vi "Run Tests Programmatically.vi"(4 "Verbose":bool=TRUE, 5 "Silent":bool, 6 "Interactive":bool=TRUE, 7 "Inspect Recursively":bool=TRUE, 9 "Report name":string, 10 "Output Folder":path, 11 "Source Folder":path) -> ()   [LabVIEW 2013]
uses:
  classes/Test Runner/Test Runner.lvclass
  classes/Test Runner/Test Runner.lvclass/Test Runner.ctl
  <userlib>/_OpenG.lib/file/file.llb/Valid Path - Traditional__ogtk.vi
  <userlib>/_OpenG.lib/file/file.llb/File Exists - Scalar__ogtk.vi
  <userlib>/_OpenG.lib/array/array.llb/Delete Elements from 1D Array (Path)__ogtk.vi
  <userlib>/_OpenG.lib/file/file.llb/Strip Path - Arrays__ogtk.vi
  <userlib>/_OpenG.lib/file/file.llb/Strip Path Extension - 1D Array of Strings__ogtk.vi
  <userlib>/_OpenG.lib/file/file.llb/Strip Path Extension - String__ogtk.vi
  <userlib>/_OpenG.lib/file/file.llb/Convert File Extension (String)__ogtk.vi
  classes/Test Report.JUnit/Test Report.JUnit.lvclass
  classes/Test Report.Default/Test Report.Default.lvclass
panel:
  in  "report format":enum16{"Plain text", "XML"}(ring)=enum."XML"
  in  "Defined Tests":i32[](listbox)
  in  "Run Batch Test":bool
  # "CARAYA Batch Testing\n\nFill in the source folder where your tests are and choose the output result options."
  # "Output Configuration"
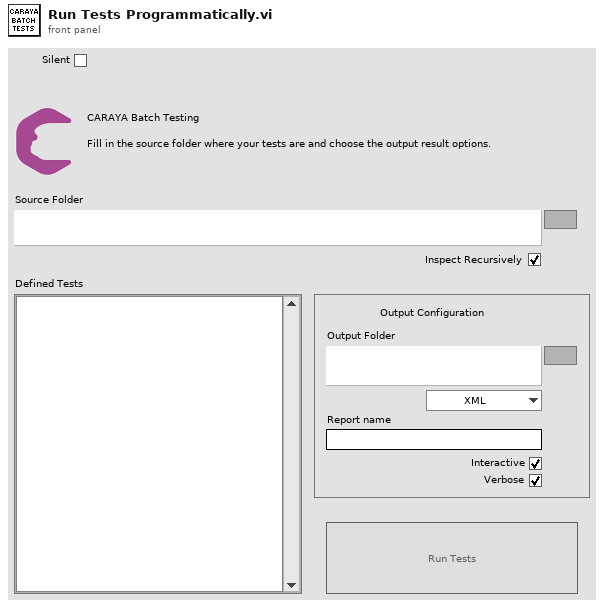
[diagram p1: front panel]
types:
  T1 = enum32{"invalid app kind", "Development System", "Run Time System", "Student Edition", "Embedded LabVIEW", "Evaluation", "Custom"}
  T2 = enum8{"Enabled", "Disabled", "Disabled and Grayed Out"}
  T3 = enum32{"Invalid", "Standard", "Closed", "Hidden", "Minimized", "Maximized"}
  T4 = cluster{"Core":cluster{"Current VI Reference":refnum<vi>, "Close Panel on Exit?":bool}, "Output Folder":path, "Report name":string, "Source Folder":path, "Interactive":bool, "Verbose":bool, "Menu Launch AppRef":refnum<vi>, "Silent":bool, "report format":enum16{"Plain text", "XML"}, "Test Runner":refnum<class "Test Runner.lvclass">}
  T5 = cluster{"Current VI Reference":refnum<vi>, "Close Panel on Exit?":bool}
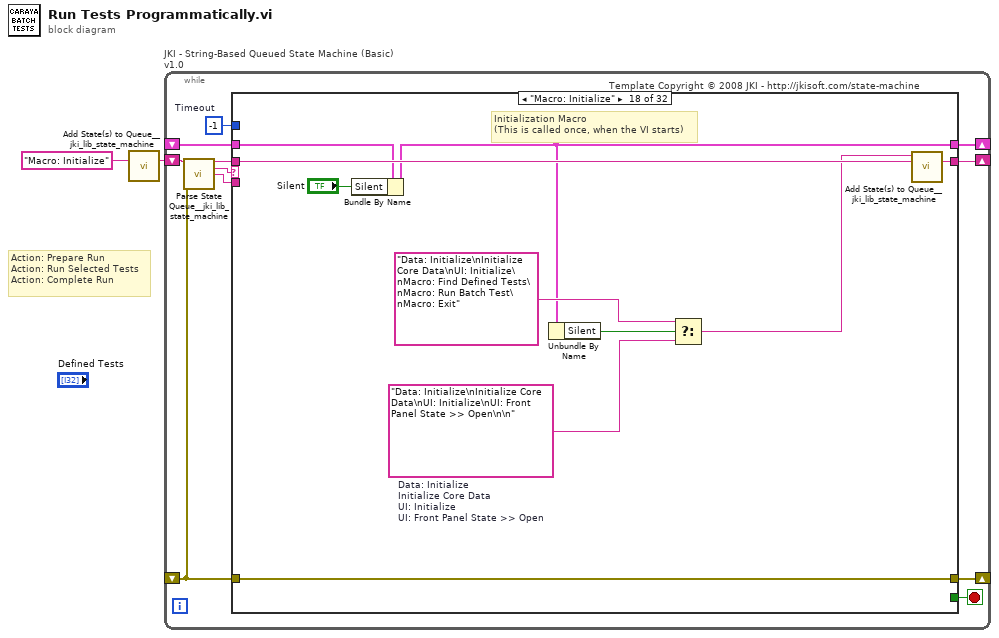
[diagram p0: block diagram]
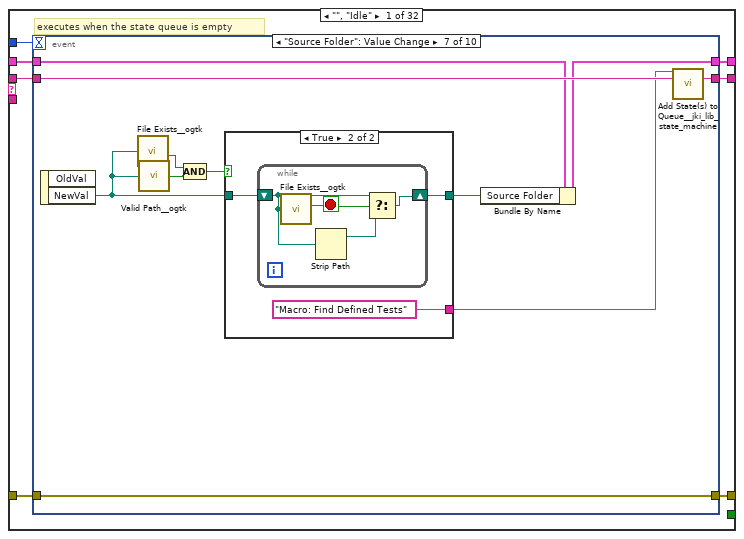
[diagram p2: hidden frame]
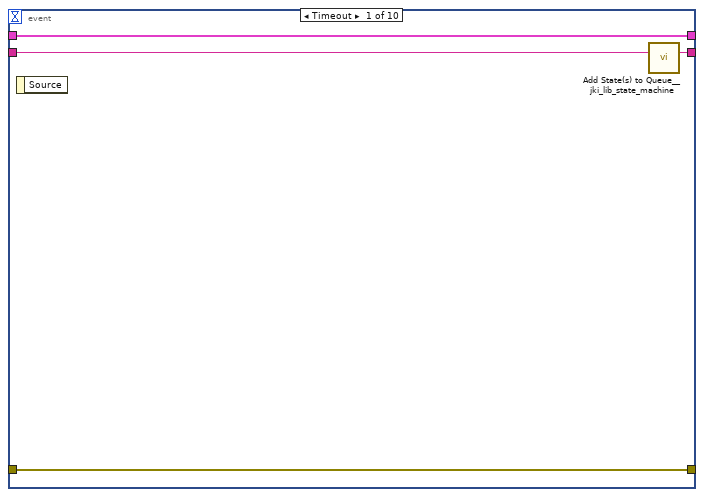
[diagram p3: hidden frame]
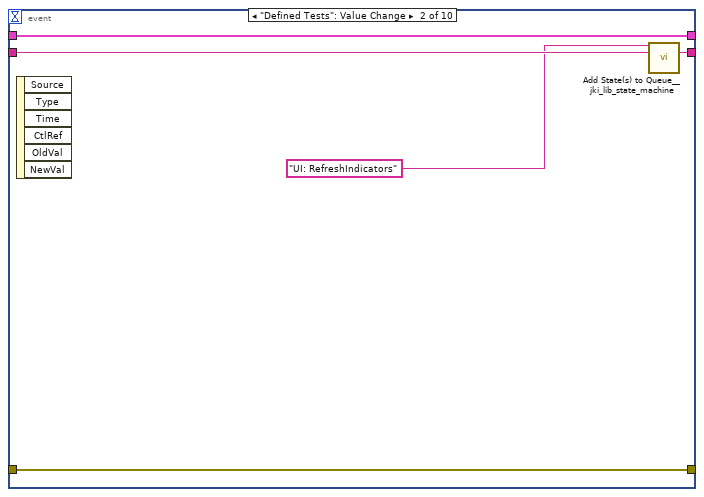
[diagram p4: hidden frame]
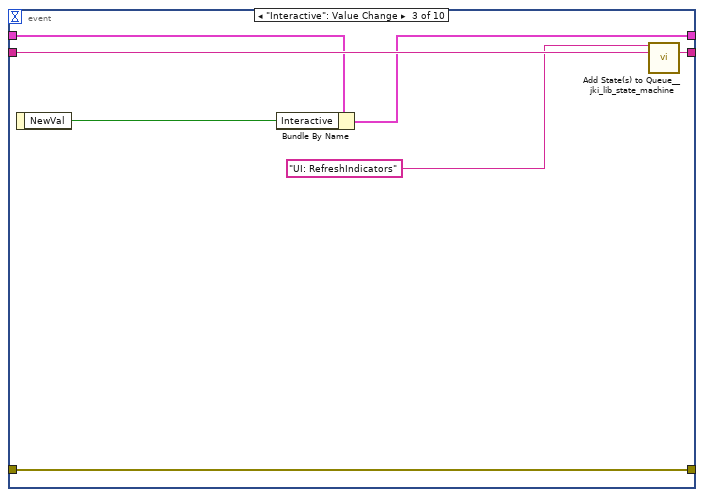
[diagram p5: hidden frame]
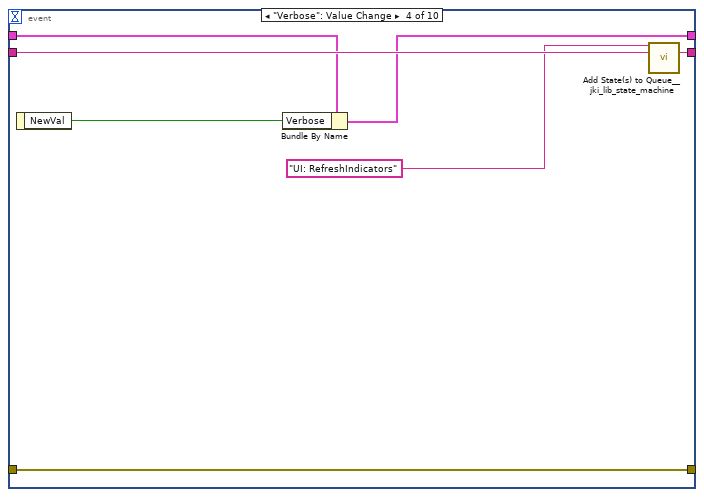
[diagram p6: hidden frame]
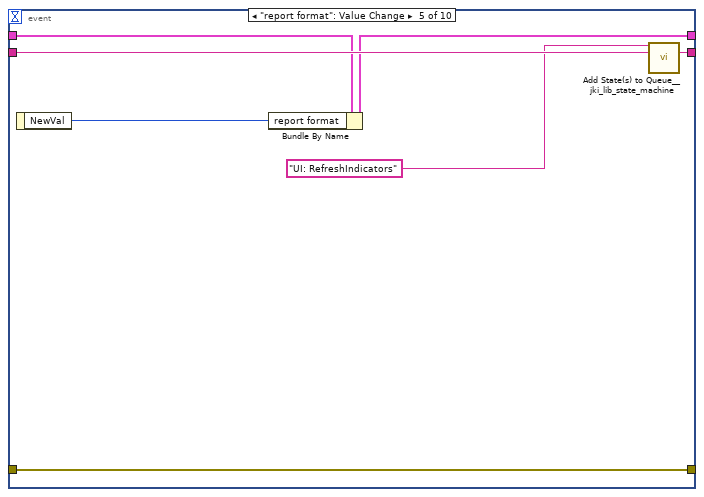
[diagram p7: hidden frame]
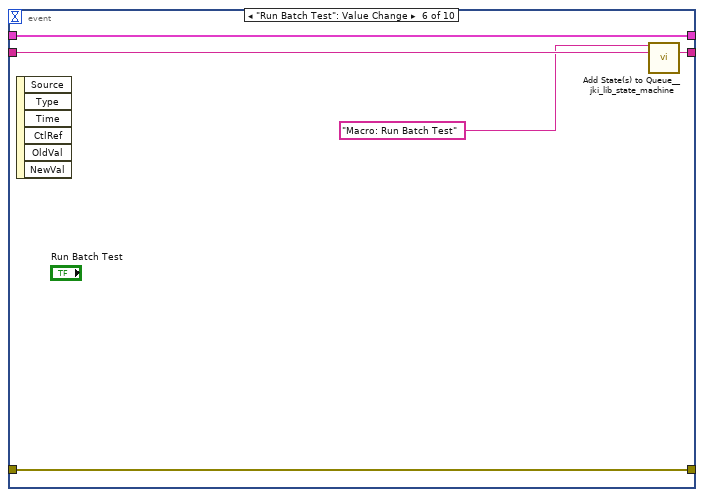
[diagram p8: hidden frame]
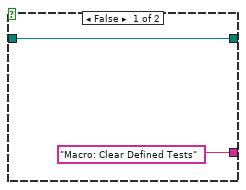
[diagram p9: hidden frame]
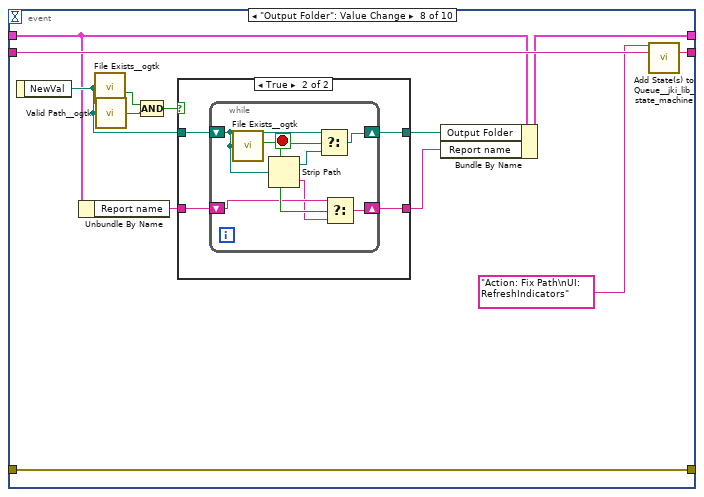
[diagram p10: hidden frame]
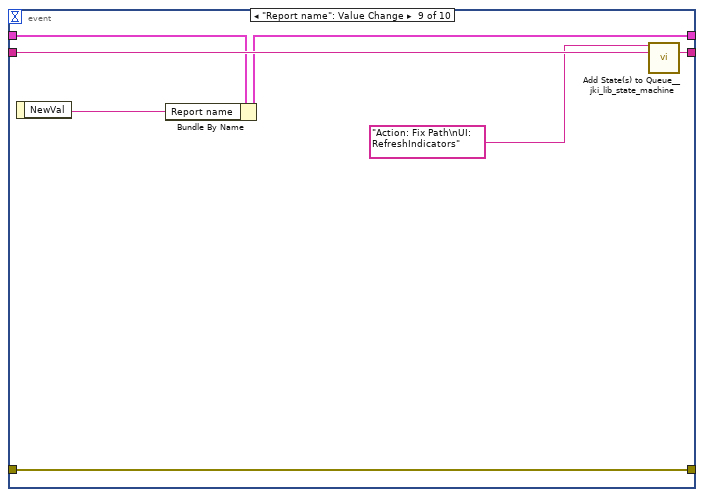
[diagram p12: hidden frame]
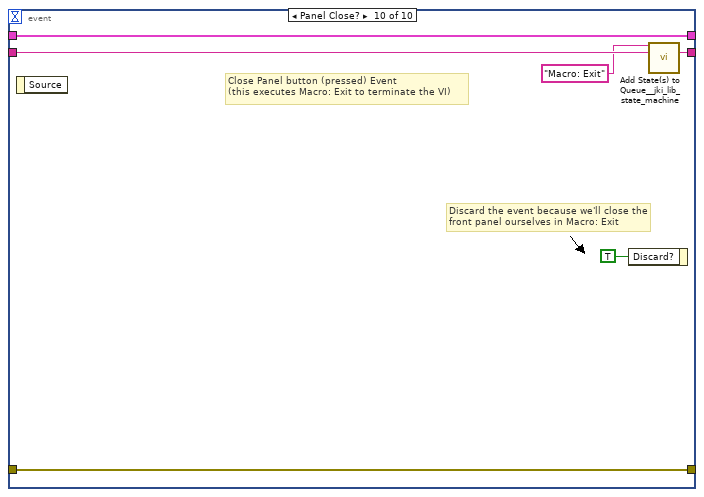
[diagram p13: hidden frame]
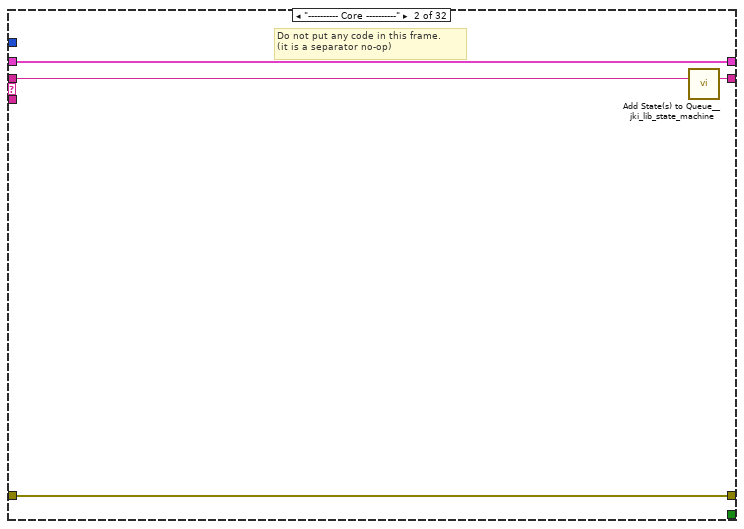
[diagram p14: hidden frame]
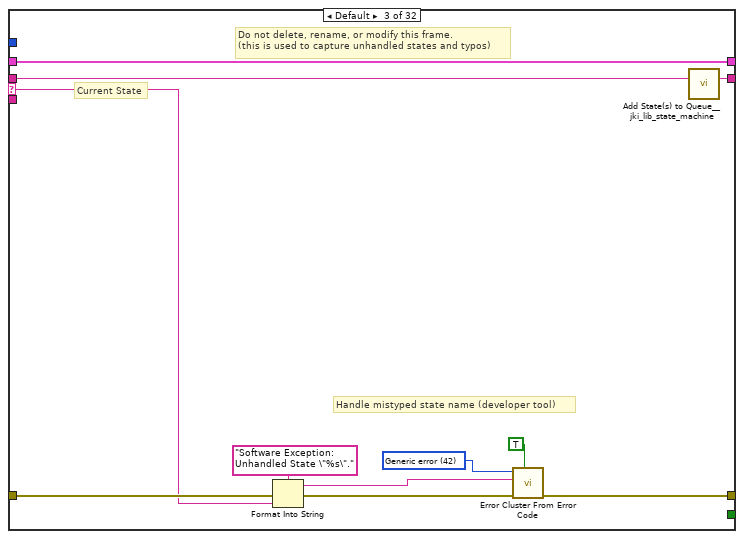
[diagram p15: hidden frame]
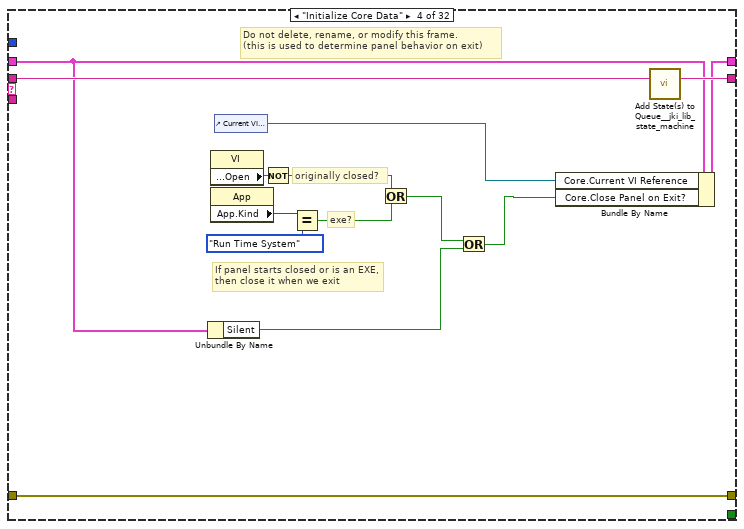
[diagram p16: hidden frame]
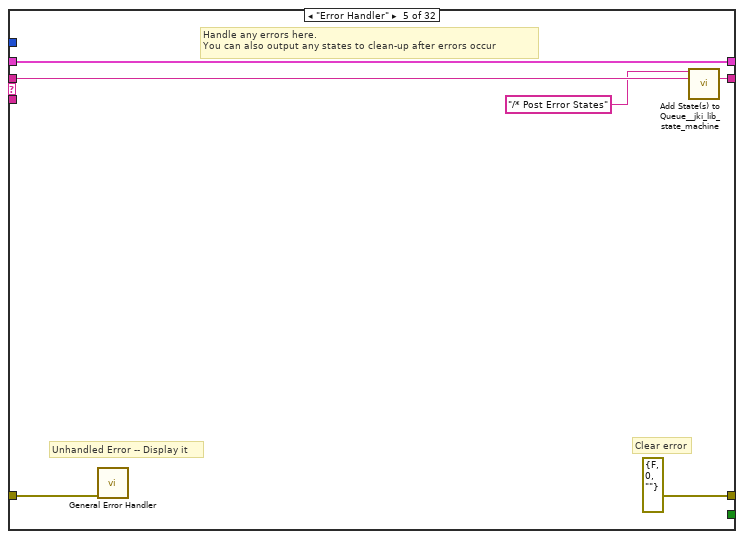
[diagram p17: hidden frame]
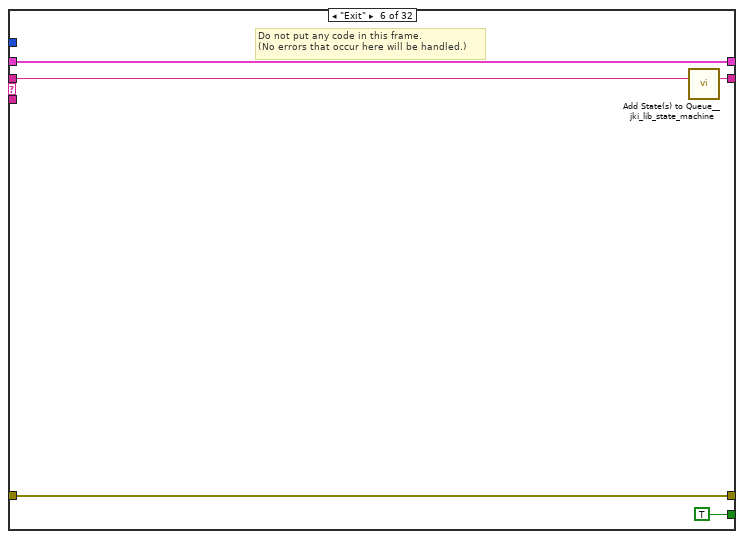
[diagram p18: hidden frame]
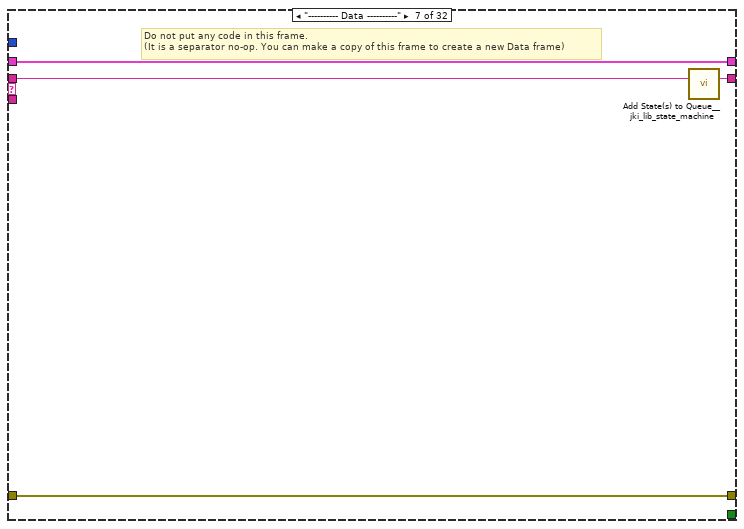
[diagram p19: hidden frame]
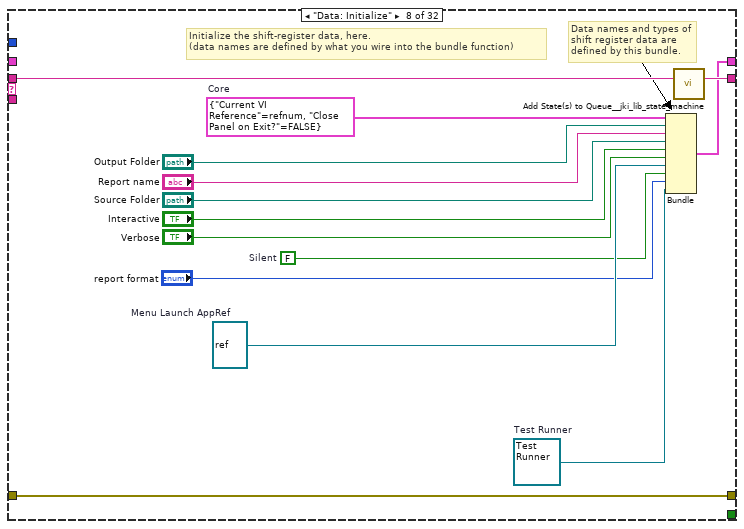
[diagram p20: hidden frame]
diagram:
  # "Action: Prepare Run\nAction: Run Selected Tests\nAction: Complete Run"
  n1 = call <vilib>:"Add State(s) to Queue__jki_lib_state_machine.vi"("State(s) in (\"\")"="Macro: Initialize") -> ("States Out"=w2:string)  [unwired: 14 in]
  n2 = while "JKI - String-Based Queued State Machine (Basic) v1.0" {
    shift-right: [w6] -> _
    shift-left: _ -> [w5]
    shift-right: [w9] -> _
    shift-left: _ -> [w3]
    shift-right: [w8] -> _
    shift-left: w2 -> [w10]
    stop <- w7 stop-if-true
    w4 = -1  # Timeout
    # "Template Copyright © 2008 JKI - http://jkisoft.com/state-machine"
    n3 = call <vilib>:"Parse State Queue__jki_lib_state_machine.vi"("State Queue"=w10, "Error In (no error)"=w3) -> ("Remaining States"=w12:string, "Current State"=w13:string, "Arguments"=w11:string)  [unwired: 11 in]
    n4 = case shown="\"Macro: Initialize\"" w13 {
      selector: w13 -> [_ _ w119 _ _ _ _ _ _ _ _ _ _ _ _ _ _ _ _ _ _ _ _ _ _ _ _ _ _ _ _ _]
      tunnel: w12 -> [w20 w118 w123 w143 w149 w154 w158 w172 w178 w182 w191 w221 w240 w251 w260 w271 w297 w307 w312 w317 w322 w327 w332 w339 w343 w361 w396 w407 w421 w428 w447 w467]
      tunnel: w11 -> [_ _ _ _ _ _ _ _ _ _ _ _ _ _ w255 w265 _ _ _ _ _ _ _ _ _ _ _ _ _ _ _ _]
      tunnel: w5 -> [w18 w115 w121 w133 w146 w152 w155 _ w173 w179 w187 w215 w238 w249 w258 w267 w294 w301 w309 w314 w319 w324 w329 w336 w340 w358 w394 w405 w415 w425 w435 w464]
      tunnel: [w17 w116 w125 w140 errorcluster {"status"=FALSE, "code"=0, "source"=""} ("error out") w151 w156 w169 w174 w180 w189 w219 w224 w244 w256 w268 w295 w305 w310 w315 w320 w325 w330 w337 w341 w359 w386 w397 w418 w426 w439 w465] -> w9
      tunnel: w3 -> [w16 w116 w124 w140 w145 w151 w156 w169 w175 w180 w189 w219 w224 w245 w257 w269 w295 w305 w310 w315 w320 w325 w330 w337 w341 w359 w387 w398 w419 w426 w440 w465]
      tunnel: [w19 w117 w122 w142 w148 w153 w157 w171 w177 w181 w190 w220 w239 w250 w259 w270 w296 w306 w311 w316 w321 w326 w331 w338 w342 w360 w395 w406 w420 w427 w446 w466] -> w8
      tunnel: [_ _ _ _ _ TRUE _ _ _ _ _ _ _ _ _ _ _ _ _ _ _ _ _ _ _ _ _ _ _ _ _ _] -> w7
      tunnel: [w15 w115 w121 w141 w146 w152 w155 w170 w173 w179 w186 w214 w237 w249 w258 w267 w294 w300 w309 w314 w319 w324 w329 w336 w340 w352 w393 w404 w414 w425 w441 w464] -> w6
      tunnel: w4 -> [w14 _ _ _ _ _ _ _ _ _ _ _ _ _ _ _ _ _ _ _ _ _ _ _ _ _ _ _ _ _ _ _]
      frame "", "Idle" {
        # "executes when the state queue is empty"
        n5 = event shown="[6] \"Source Folder\": Value Change" {
          selector: _ -> [_ _ _ _ _ _ _ _ _ _]
          dyn-events: _ -> [_ _ _ _ _ _ _ _ _ _]
          timeout: w14 -> [_ _ _ _ _ _ _ _ _ _]
          tunnel: w20 -> [w24 w29 w36 w43 w50 w55 w66 w88 w108 w114]
          tunnel: [w23 w28 w35 w42 w49 w54 w65 w87 w107 w113] -> w19
          tunnel: w18 -> [w21 w26 w31 w38 w45 w52 w63 w78 w105 w111]
          tunnel: [w22 w27 w34 w41 w48 w53 w64 w86 w106 w112] -> w17
          tunnel: w16 -> [w22 w27 w34 w41 w48 w53 w64 w86 w106 w112]
          tunnel: [w21 w26 w30 w37 w44 w52 w62 w85 w104 w111] -> w15
          event Timeout {
            n6 = event-data() -> ()  [unwired: 1 in, 1 out]
            n7 = call <vilib>:"Add State(s) to Queue__jki_lib_state_machine.vi"("State(s) in (\"\")"=w24) -> ("States Out"=w23:string)  [unwired: 14 in]
          }
          event "Defined Tests": Value Change {
            n8 = event-data() -> ()  [unwired: 1 in, 6 out]
            n9 = call <vilib>:"Add State(s) to Queue__jki_lib_state_machine.vi"("State(s) in Front (\"\")"="UI: RefreshIndicators", "State(s) in (\"\")"=w29) -> ("States Out"=w28:string)  [unwired: 13 in]
          }
          event "Interactive": Value Change {
            n10 = event-data() -> ("NewVal"=w32:bool)  [unwired: 1 in]
            n11 = Bundle By Name(cluster=w31, "Interactive"=w32) -> (w30:T4)
            n12 = call <vilib>:"Add State(s) to Queue__jki_lib_state_machine.vi"("State(s) in Front (\"\")"="UI: RefreshIndicators", "State(s) in (\"\")"=w36) -> ("States Out"=w35:string)  [unwired: 13 in]
          }
          event "Verbose": Value Change {
            n13 = event-data() -> ("NewVal"=w39:bool)  [unwired: 1 in]
            n14 = Bundle By Name(cluster=w38, "Verbose"=w39) -> (w37:T4)
            n15 = call <vilib>:"Add State(s) to Queue__jki_lib_state_machine.vi"("State(s) in Front (\"\")"="UI: RefreshIndicators", "State(s) in (\"\")"=w43) -> ("States Out"=w42:string)  [unwired: 13 in]
          }
          event "report format": Value Change {
            n16 = event-data() -> ("NewVal"=w46:enum16{"Plain text", "XML"})  [unwired: 1 in]
            n17 = Bundle By Name(cluster=w45, "report format"=w46) -> (w44:T4)
            n18 = call <vilib>:"Add State(s) to Queue__jki_lib_state_machine.vi"("State(s) in Front (\"\")"="UI: RefreshIndicators", "State(s) in (\"\")"=w50) -> ("States Out"=w49:string)  [unwired: 13 in]
          }
          event "Run Batch Test": Value Change {
            n19 = event-data() -> ()  [unwired: 1 in, 6 out]
            n20 = call <vilib>:"Add State(s) to Queue__jki_lib_state_machine.vi"("State(s) in Front (\"\")"="Macro: Run Batch Test", "State(s) in (\"\")"=w55) -> ("States Out"=w54:string)  [unwired: 13 in]
          }
          event "Source Folder": Value Change {
            n21 = event-data() -> ("NewVal"=w58:path)  [unwired: 1 in, 1 out]
            n22 = call-poly <userlib>:"File Exists__ogtk.vi"("file path"=w58) -> ("exists"=w60:bool)  [unwired: 6 in, 1 out]
            n23 = call-poly <userlib>:"Valid Path__ogtk.vi"("path"=w58) -> ("valid"=w61:bool)
            n24 = Compound Arithmetic op=AND(w60, w61) -> (w59:bool)
            n25 = case shown="True" w59 {
              tunnel: w58 -> [w68 w71]
              tunnel: [w68 w70] -> w57
              tunnel: ["Macro: Clear Defined Tests" "Macro: Find Defined Tests"] -> w56
              frame False {
              }
              frame True {
                n26 = while {
                  shift-right: [w74] -> w70
                  shift-left: w71 -> [w73]
                  stop <- w75 stop-if-true
                  n27 = call-poly <userlib>:"File Exists__ogtk.vi"("file path"=w73) -> ("is directory"=w75:bool)  [unwired: 6 in, 1 out]
                  n28 = Strip Path(path=w73) -> (stripped path=w72:path)  [unwired: 1 out]
                  n29 = Select(t=w73, s=w75, f=w72) -> (s? t:f=w74:path)
                }
              }
            }
            n30 = Bundle By Name(cluster=w63, "Source Folder"=w57) -> (w62:T4)
            n31 = call <vilib>:"Add State(s) to Queue__jki_lib_state_machine.vi"("State(s) in Front (\"\")"=w56, "State(s) in (\"\")"=w66) -> ("States Out"=w65:string)  [unwired: 13 in]
          }
          event "Output Folder": Value Change {
            n32 = event-data() -> ("NewVal"=w81:path)  [unwired: 1 in]
            n33 = Unbundle By Name(w78) -> ("Report name"=w77:string)
            n34 = call-poly <userlib>:"File Exists__ogtk.vi"("file path"=w81) -> ("exists"=w83:bool)  [unwired: 6 in, 1 out]
            n35 = call-poly <userlib>:"Valid Path__ogtk.vi"("path"=w81) -> ("valid"=w84:bool)
            n36 = Compound Arithmetic op=AND(w83, w84) -> (w82:bool)
            n37 = case shown="True" w82 {
              tunnel: w81 -> [w90 w94]
              tunnel: [w90 w93] -> w80
              tunnel: w77 -> [w89 w92]
              tunnel: [w89 w91] -> w76
              frame False {
              }
              frame True {
                n38 = while {
                  shift-right: [w101] -> w93
                  shift-left: w94 -> [w100]
                  shift-right: [w95] -> w91
                  shift-left: w92 -> [w97]
                  stop <- w98 stop-if-true
                  n39 = call-poly <userlib>:"File Exists__ogtk.vi"("file path"=w100) -> ("is directory"=w98:bool)  [unwired: 6 in, 1 out]
                  n40 = Strip Path(path=w100) -> (stripped path=w99:path, name=w96:string)
                  n41 = Select(t=w100, s=w98, f=w99) -> (s? t:f=w101:path)
                  n42 = Select(t=w97, s=w98, f=w96) -> (s? t:f=w95:string)
                }
              }
            }
            n43 = Bundle By Name(cluster=w78, "Output Folder"=w80, "Report name"=w76) -> (w85:T4)
            n44 = call <vilib>:"Add State(s) to Queue__jki_lib_state_machine.vi"("State(s) in Front (\"\")"="Action: Fix Path\nUI: RefreshIndicators", "State(s) in (\"\")"=w88) -> ("States Out"=w87:string)  [unwired: 13 in]
          }
          event "Report name": Value Change {
            n45 = event-data() -> ("NewVal"=w103:string)  [unwired: 1 in]
            n46 = Bundle By Name(cluster=w105, "Report name"=w103) -> (w104:T4)
            n47 = call <vilib>:"Add State(s) to Queue__jki_lib_state_machine.vi"("State(s) in Front (\"\")"="Action: Fix Path\nUI: RefreshIndicators", "State(s) in (\"\")"=w108) -> ("States Out"=w107:string)  [unwired: 13 in]
          }
          event Panel Close? {
            # "Discard the event because we'll close the front panel ourselves in Macro: Exit"
            # "Close Panel button (pressed) Event\n(this executes Macro: Exit to terminate the VI)"
            n48 = event-data() -> ()  [unwired: 1 in, 1 out]
            n49 = event-data("Discard?"=TRUE) -> ()  [unwired: 1 in, 1 out]
            n50 = call <vilib>:"Add State(s) to Queue__jki_lib_state_machine.vi"("State(s) in Front (\"\")"="Macro: Exit", "State(s) in (\"\")"=w114) -> ("States Out"=w113:string)  [unwired: 13 in]
          }
        }
      }
      frame "---------- Core ----------" {
        # "Do not put any code in this frame.\n(it is a separator no-op)"
        n51 = call <vilib>:"Add State(s) to Queue__jki_lib_state_machine.vi"("State(s) in (\"\")"=w118) -> ("States Out"=w117:string)  [unwired: 14 in]
      }
      frame Default {
        w128 = 42 items=["No error", "Argument error", "Memory is full", "Out of zone", "End of file", "File already open", "Generic file I/O error", "File not found", "File permission error", "Disk is full", "Duplicate path", "Too many files open", "System feature not enabled", "Resource file not found", "Cannot add resource", "Resource not found", "Image not found", "Image memory error", "Pen does not exist", "Config type invalid", "Config token not found", "Config parse error", "Config memory error", "Bad external code format", "Bad external code offset", "External code not present", "Null window", "Destroy window error", "Null menu", "Print aborted", "Bad print record", "Print driver error", "Windows error during printing", "Memory error during printing", "Print dialog error", "Generic print error", "Invalid device refnum", "Device not found", "Device parameter error", "Device unit error", "Cannot open device", "Device call aborted", "Generic error", "Cancelled by user", "Object ID too low", "Object ID too high", "Object not in heap", "Unknown heap", "Unknown object (invalid DefProc)", "Unknown object (DefProc not in table)", "Message out of range", "Invalid (null) method", "Unknown message", "Manager call not supported", "Bad address", "Network operation in progress", "Network operation timed out", "Connection is busy", "Network attribute not supported", "Network error", "Address in use", "System out of memory", "Connection aborted", "Connection refused", "Not connected", "Already connected", "Connection closed", "Initialization error (interapplication manager)", "Bad occurrence", "Wait on unbound occurrence handler", "Occurrence queue overflow", "Datalog type conflict", "Unused", "Unrecognized type (interapplication manager)", "Memory corrupt", "Failed to make temporary DLL", "Old CIN version", "Drag socket not found", "Failed to load drop-object", "Failed to register OLE object", "Failed to release OLE object", "Format specifier type mismatch", "Unknown format specifier", "Too few format specifiers", "Too many format specifiers", "Scan failed", "Newer CIN version", "Error converting to variant", "Runtime menu error", "Password tampered", "Variant attribute not found", "Incompatible variant data type", "Event data is not available", "Event Store is not present", "Occurrence is not found", "Event Queue is not created", "Event info is not available", "Refnum passed is NULL", "Error retrieving Class GUID", "Error retrieving CoClass GUID", "Error retrieving TypeLib GUID.", "Bad built application magic bytes.", "Specific driver is different from the specific driver associated with the Logical Name.", "There is no session opened to the class driver.", "Max Error", "MAX - Error with config objects", "MAX - Error loading configuration", "MAX - Group not supported"]
        # "Current State"
        # "Do not delete, rename, or modify this frame.\n(this is used to capture unhandled states and typos)"
        # "Handle mistyped state name (developer tool)"
        n52 = Format Into String(format string="Software Exception: Unhandled State \"%s\"." ("message"), error in=w124, w119) -> (resulting string=w127:string, error out=w126:errorcluster)  [unwired: 1 in]
        n53 = call <vilib>:"Error Cluster From Error Code.vi"("show call chain? (False)"=TRUE, "error in (no error)"=w126, "error message (\"\")"=w127, "error code (0)"=w128) -> ("error out"=w125:errorcluster)  [unwired: 5 in]
        n54 = call <vilib>:"Add State(s) to Queue__jki_lib_state_machine.vi"("State(s) in (\"\")"=w123) -> ("States Out"=w122:string)  [unwired: 14 in]
      }
      frame "Initialize Core Data" {
        # "Do not delete, rename, or modify this frame.\n(this is used to determine panel behavior on exit)"
        # "originally closed?"
        # "exe?"
        # "If panel starts closed or is an EXE, then close it when we exit"
        n55 = Unbundle By Name(w133) -> ("Silent"=w132:bool)
        n56 = property class="VI"() -> ("Front Panel.Open"=w139:bool)  [unwired: 2 in, 2 out]
        n57 = property class="App"() -> ("App.Kind"=w138:T1)  [unwired: 2 in, 2 out]
        n58 = control-ref of="Current VI Reference"() -> (w134:refnum<vi>)
        n59 = Not(x=w139) -> (.not. x?=w136:bool)
        n60 = Equal?(x=w138, y=T1."Run Time System" ("Application:Kind")) -> (x = y?=w135:bool)
        n61 = Or(x=w136, y=w135) -> (x .or. y?=w131:bool)
        n62 = Or(x=w131, y=w132) -> (x .or. y?=w130:bool)
        n63 = Bundle By Name(cluster=w133, "Core.Current VI Reference"=w134, "Core.Close Panel on Exit?"=w130) -> (w141:T4)
        n64 = call <vilib>:"Add State(s) to Queue__jki_lib_state_machine.vi"("State(s) in (\"\")"=w143) -> ("States Out"=w142:string)  [unwired: 14 in]
      }
      frame "Error Handler" {
        # "Unhandled Error -- Display it"
        # "Handle any errors here.\nYou can also output any states to clean-up after errors occur"
        # "Clear error"
        n65 = call <vilib>:"General Error Handler.vi"("error in (no error)"=w145) -> ()  [unwired: 10 in, 5 out]
        n66 = call <vilib>:"Add State(s) to Queue__jki_lib_state_machine.vi"("State(s) in Front (\"\")"="/* Post Error States", "State(s) in (\"\")"=w149) -> ("States Out"=w148:string)  [unwired: 13 in]
      }
      frame "Exit" {
        # "Do not put any code in this frame.\n(No errors that occur here will be handled.)"
        n67 = call <vilib>:"Add State(s) to Queue__jki_lib_state_machine.vi"("State(s) in (\"\")"=w154) -> ("States Out"=w153:string)  [unwired: 14 in]
      }
      frame "---------- Data ----------" {
        # "Do not put any code in this frame.\n(It is a separator no-op. You can make a copy of this frame to create a new Data frame)"
        n68 = call <vilib>:"Add State(s) to Queue__jki_lib_state_machine.vi"("State(s) in (\"\")"=w158) -> ("States Out"=w157:string)  [unwired: 14 in]
      }
      frame "Data: Initialize" {
        w159 = FALSE  # Silent
        w160 = refnum<class "Test Runner.lvclass"> refnum  # Test Runner
        w167 = refnum<vi> refnum  # Menu Launch AppRef
        w168 = T5 {"Current VI Reference"=refnum, "Close Panel on Exit?"=FALSE}  # Core
        # "Data names and types of shift register data are defined by this bundle."
        # "Initialize the shift-register data, here.\n(data names are defined by what you wire into the bundle function)"
        n69 = Bundle("Core"=w168, "Output Folder"="Output Folder", "Report name"="Report name", "Source Folder"="Source Folder", "Interactive"="Interactive", "Verbose"="Verbose", "Menu Launch AppRef"=w167, "Silent"=w159, "report format"="report format", "Test Runner"=w160) -> (w170:T4)  [unwired: 1 in]
        n70 = call <vilib>:"Add State(s) to Queue__jki_lib_state_machine.vi"("State(s) in (\"\")"=w172) -> ("States Out"=w171:string)  [unwired: 14 in]
      }
      frame "Data: Cleanup" {
        # "Cleanup any data and references, here.\n(this is called automatically, by the Macro: Exit)"
        n71 = Unbundle By Name(w173) -> ("Core.Current VI Reference"=w176:refnum<vi>)
        n72 = Close Reference(reference=w176, error in (no error)=w175) -> (error out=w174:errorcluster)
        n73 = call <vilib>:"Add State(s) to Queue__jki_lib_state_machine.vi"("State(s) in (\"\")"=w178) -> ("States Out"=w177:string)  [unwired: 14 in]
      }
      frame "---------- UI ----------" {
        # "Do not put any code in this frame.\n(It is a separator no-op. You can make a copy of this frame to create a new UI frame)"
        n74 = call <vilib>:"Add State(s) to Queue__jki_lib_state_machine.vi"("State(s) in (\"\")"=w182) -> ("States Out"=w181:string)  [unwired: 14 in]
      }
      frame "UI: Initialize" {
        # "If Silent, do not set\ninteractive flag to True"
        # "Initialize the User Interface, here.\n(this is called automatically, by the Macro: Init)"
        n75 = Unbundle By Name(w187) -> ("Interactive"=w185:bool, "Silent"=w184:bool)
        n76 = Compound Arithmetic op=AND(w185, invert w184) -> (w183:bool)
        n77 = Bundle By Name(cluster=w187, "Interactive"=w183) -> (w186:T4)
        n78 = call <vilib>:"Add State(s) to Queue__jki_lib_state_machine.vi"("State(s) in Front (\"\")"="UI: Refresh Defined Tests\nAction: Fix Path\nUI: Initialize Path\nUI: RefreshIndicators" ("Text.Text"), "State(s) in (\"\")"=w191) -> ("States Out"=w190:string)  [unwired: 13 in]
      }
      frame "UI: RefreshIndicators" {
        n79 = Unbundle By Name(w215) -> ("Report name"=w194:string, "Output Folder"=w195:path, "Interactive"=w213:bool, "Source Folder"=w204:path, "report format"=w192:enum16{"Plain text", "XML"}, "Test Runner"=w205:refnum<class "Test Runner.lvclass">)
        n80 = property on="Defined Tests" class="LstBox (strict)"() -> ("Value"=w193:i32[])  [unwired: 2 in, 2 out]
        n81 = local write "Output Folder"(w195) -> ()
        n82 = local write "Report name"(w194) -> ()
        n83 = local write "Source Folder"(w204) -> ()
        n84 = local write "report format"(w192) -> ()
        n85 = call-dynamic "Read Test VIs.vi"("Test Runner in"=w205) -> ("Test VIs"=w200:path[], "Test Runner out"=w201:refnum<class "Test Runner.lvclass">)  [unwired: 8 in, 1 out]
        n86 = Empty Array?(array=w200) -> (empty?=w199:bool)
        n87 = Empty Array?(array=w193) -> (empty?=w202:bool)
        n88 = call-poly <userlib>:"Delete Elements from Array__ogtk.vi"("indices"=w193, "array"=w200) -> ("array w/ subset deleted"=w198:path[])  [unwired: 8 in, 1 out]
        n89 = Array Size(array=w193) -> (size(s)=w208:i32)
        n90 = Select(t=path[] [], s=w199, f=w198) -> (s? t:f=w197:path[])
        n91 = Format Into String(format string="Run Selected Tests (%d)", w208) -> (resulting string=w206:string)  [unwired: 2 in, 1 out]
        n92 = call "Write Excluded Tests.vi"("Excluded Tests"=w197, "Test Runner in"=w201) -> ("Test Runner out"=w203:refnum<class "Test Runner.lvclass">)  [unwired: 8 in, 1 out]
        n93 = Select(t="Run All Tests", s=w202, f=w206) -> (s? t:f=w210:string)
        n94 = Bundle By Name(cluster=w215, "Interactive"=w213, "Test Runner"=w203) -> (w214:T4)
        n95 = Select(t="Run Tests", s=w199, f=w210) -> (s? t:f=w211:string)
        n96 = Select(t=T2."Disabled and Grayed Out" ("Disabled"), s=w199, f=T2."Enabled" ("Disabled")) -> (s? t:f=w216:T2)
        n97 = property on="Run Batch Test" class="Bool"("BoolText.Text"=w211) -> ()  [unwired: 2 in, 2 out]
        n98 = property on="Run Batch Test" class="Bool"("DisabledEnum"=w216) -> ()  [unwired: 2 in, 2 out]
        n99 = call <vilib>:"Add State(s) to Queue__jki_lib_state_machine.vi"("State(s) in (\"\")"=w221) -> ("States Out"=w220:string)  [unwired: 14 in]
      }
      frame "UI: Initialize Path" {
        n100 = Unbundle By Name(w238) -> ("Source Folder"=w231:path, "Output Folder"=w225:path)  [unwired: 1 out]
        n101 = call-poly <userlib>:"Valid Path__ogtk.vi"("path"=w225) -> ("valid"=w228:bool)
        n102 = call-poly <userlib>:"File Exists__ogtk.vi"("file path"=w225) -> ("is directory"=w226:bool, "exists"=w227:bool)  [unwired: 6 in]
        n103 = call-poly <userlib>:"Valid Path__ogtk.vi"("path"=w231) -> ("valid"=w234:bool)
        n104 = call-poly <userlib>:"File Exists__ogtk.vi"("file path"=w231) -> ("is directory"=w236:bool, "exists"=w235:bool)  [unwired: 6 in]
        n105 = Compound Arithmetic op=AND(w226, w227, w228) -> (w229:bool)
        n106 = Compound Arithmetic op=AND(w236, w235, w234) -> (w233:bool)
        n107 = Select(t=w225, s=w229, f=path "") -> (s? t:f=w222:path)
        n108 = Select(t=w231, s=w233, f=path "") -> (s? t:f=w230:path)
        n109 = Bundle By Name(cluster=w238, "Source Folder"=w230, "Output Folder"=w222) -> (w237:T4)
        n110 = call <vilib>:"Add State(s) to Queue__jki_lib_state_machine.vi"("State(s) in (\"\")"=w240) -> ("States Out"=w239:string)  [unwired: 14 in]
      }
      frame "UI: Refresh Defined Tests" {
        n111 = Unbundle By Name(w249) -> ("Test Runner"=w247:refnum<class "Test Runner.lvclass">)
        n112 = call-dynamic "Read Test VIs.vi"("error in (no error)"=w245, "Test Runner in"=w247) -> ("error out"=w244:errorcluster, "Test VIs"=w246:path[])  [unwired: 7 in, 1 out]
        n113 = call-poly <userlib>:"Strip Path__ogtk.vi"("path"=w246) -> ("name"=w248:string[])  [unwired: 1 out]
        n114 = property on="Defined Tests" class="LstBox (strict)"() -> ("Item Names"=w242:string[])  [unwired: 2 in, 2 out]
        n115 = call-poly <userlib>:"Strip Path Extension__ogtk.vi"("paths"=w248) -> ("roots"=w243:string[])  [unwired: 1 out]
        n116 = Not Equal?(x=w243, y=w242) -> (x != y?=w241:bool)
        n117 = case shown="True" w241 {
          tunnel: w243 -> [_ w254]
          frame False {
          }
          frame True {
            n118 = property on="Defined Tests" class="LstBox (strict)"("Item Names"=w254, "Value"=i32[] [] ("Defined Tests"), "Top Row"=0) -> ()  [unwired: 2 in, 2 out]
          }
        }
        n119 = call <vilib>:"Add State(s) to Queue__jki_lib_state_machine.vi"("State(s) in (\"\")"=w251) -> ("States Out"=w250:string)  [unwired: 14 in]
      }
      frame "UI: Cursor Set" {
        # "Argument"
        # "Set and Unset Cursor Busy.\n(Usage: \"UI: Cursor Set >> Busy|Idle\")"
        n120 = case shown="\"Idle\", Default" w255 {
          tunnel: w257 -> [w262 w264]
          tunnel: [w261 w263] -> w256
          frame "Idle", Default {
            n121 = call <vilib>:"Unset Busy.vi"("error in (no error)"=w262) -> ("error out"=w261:errorcluster)  [unwired: 10 in]
          }
          frame "Busy" {
            n122 = call <vilib>:"Set Busy.vi"("error in (no error)"=w264) -> ("error out"=w263:errorcluster)  [unwired: 9 in, 1 out]
          }
        }
        n123 = call <vilib>:"Add State(s) to Queue__jki_lib_state_machine.vi"("State(s) in (\"\")"=w260) -> ("States Out"=w259:string)  [unwired: 14 in]
      }
      frame "UI: Front Panel State" {
        # "Argument"
        # "Set Front Panel Open or Closed\n(Usage: \"UI: Front Panel State >> Open|Close\")"
        n124 = Unbundle By Name(w267) -> ("Core.Current VI Reference"=w266:refnum<vi>)
        n125 = case shown="\"Open\", Default" w265 {
          tunnel: w269 -> [w275 w288]
          tunnel: [w277 w289] -> w268
          tunnel: w266 -> [w276 w286]
          frame "Open", Default {
            n126 = property class="VI"(reference=w276, error in=w275) -> (reference out=w273:refnum<vi>, error out=w274:errorcluster, "Front Panel.Open"=w272:bool)
            n127 = case shown="False" w272 {
              tunnel: [w280 w283] -> w277
              tunnel: w274 -> [w279 w283]
              tunnel: w273 -> [w278 _]
              frame False {
                n128 = invoke class="VI" method="FP.Open"(reference=w278, error in=w279, "Activate"=TRUE, "State"=T3."Standard") -> (error out=w280:errorcluster)  [unwired: 1 in, 4 out]
              }
              frame True {
              }
            }
          }
          frame "Close" {
            n129 = property class="VI"(reference=w286, error in=w288) -> (reference out=w285:refnum<vi>, error out=w287:errorcluster, "Front Panel.Open"=w284:bool)
            n130 = case shown="True" w284 {
              tunnel: [w290 w293] -> w289
              tunnel: w287 -> [w290 w292]
              tunnel: w285 -> [_ w291]
              frame False {
              }
              frame True {
                n131 = invoke class="VI" method="FP.Close"(reference=w291, error in=w292) -> (error out=w293:errorcluster)  [unwired: 1 in, 2 out]
              }
            }
          }
        }
        n132 = call <vilib>:"Add State(s) to Queue__jki_lib_state_machine.vi"("State(s) in (\"\")"=w271) -> ("States Out"=w270:string)  [unwired: 14 in]
      }
      frame "---------- Macro ----------" {
        # "Do not put any code in this frame.\n(It is a separator no-op. You can make a copy of this frame to create a new Macro frame)"
        n133 = call <vilib>:"Add State(s) to Queue__jki_lib_state_machine.vi"("State(s) in (\"\")"=w297) -> ("States Out"=w296:string)  [unwired: 14 in]
      }
      frame "Macro: Initialize" {
        w304 = "Data: Initialize\nInitialize Core Data\nUI: Initialize\nUI: Front Panel State >> Open\n\n"  # Data: Initialize Initialize Core Data UI: Initialize UI: Front Panel State >> Open
        # "Initialization Macro\n(This is called once, when the VI starts)"
        n134 = Bundle By Name(cluster=w301, "Silent"="Silent") -> (w300:T4)
        n135 = Unbundle By Name(w300) -> ("Silent"=w298:bool)
        n136 = Select(t="Data: Initialize\nInitialize Core Data\nUI: Initialize\nMacro: Find Defined Tests\nMacro: Run Batch Test\nMacro: Exit", s=w298, f=w304) -> (s? t:f=w302:string)
        n137 = call <vilib>:"Add State(s) to Queue__jki_lib_state_machine.vi"("State(s) in Front (\"\")"=w302, "State(s) in (\"\")"=w307) -> ("States Out"=w306:string)  [unwired: 13 in]
      }
      frame "Macro: ComputePath" {
        n138 = call <vilib>:"Add State(s) to Queue__jki_lib_state_machine.vi"("State(s) in Front (\"\")"="UI: RefreshIndicators", "State(s) in (\"\")"=w312) -> ("States Out"=w311:string)  [unwired: 13 in]
      }
      frame "Macro: AppendClassName" {
        n139 = call <vilib>:"Add State(s) to Queue__jki_lib_state_machine.vi"("State(s) in Front (\"\")"="UI: RefreshIndicators", "State(s) in (\"\")"=w317) -> ("States Out"=w316:string)  [unwired: 13 in]
      }
      frame "Macro: Find Defined Tests" {
        n140 = call <vilib>:"Add State(s) to Queue__jki_lib_state_machine.vi"("State(s) in Front (\"\")"="Action: Find All Defined Tests\nUI: Refresh Defined Tests\nUI: RefreshIndicators", "State(s) in (\"\")"=w322) -> ("States Out"=w321:string)  [unwired: 13 in]
      }
      frame "Macro: Clear Defined Tests" {
        n141 = call <vilib>:"Add State(s) to Queue__jki_lib_state_machine.vi"("State(s) in Front (\"\")"="Action: Reset\nUI: Refresh Defined Tests\nUI: RefreshIndicators", "State(s) in (\"\")"=w327) -> ("States Out"=w326:string)  [unwired: 13 in]
      }
      frame "Macro: Run Batch Test" {
        n142 = call <vilib>:"Add State(s) to Queue__jki_lib_state_machine.vi"("State(s) in Front (\"\")"="Action: Prepare Run\nAction: Run Selected Tests\nAction: Complete Run", "State(s) in (\"\")"=w332) -> ("States Out"=w331:string)  [unwired: 13 in]
      }
      frame "Macro: Exit" {
        # "Exit Macro\n(This is called once, when the VI exits)"
        n143 = Unbundle By Name(w336) -> ()  [unwired: 1 out]
        n144 = call <vilib>:"Add State(s) to Queue__jki_lib_state_machine.vi"("State(s) in Front (\"\")"="UI: Front Panel State >> Close", "State(s) at Back (\"\")"="Data: Cleanup\nExit") -> ("States Out"=w334:string)  [unwired: 13 in]
        n145 = call <vilib>:"Add State(s) to Queue__jki_lib_state_machine.vi"("State(s) in Front (\"\")"=w334, "State(s) in (\"\")"=w339) -> ("States Out"=w338:string)  [unwired: 13 in]
      }
      frame "---------- Action ----------" {
        n146 = call <vilib>:"Add State(s) to Queue__jki_lib_state_machine.vi"("State(s) in (\"\")"=w343) -> ("States Out"=w342:string)  [unwired: 14 in]
      }
      frame "Action: Fix Path" {
        n147 = Unbundle By Name(w358) -> ("Output Folder"=w354:path, "Report name"=w351:string, "report format"=w349:enum16{"Plain text", "XML"})
        n148 = call-poly <userlib>:"File Exists__ogtk.vi"("file path"=w354) -> ("exists"=w356:bool)  [unwired: 6 in, 1 out]
        n149 = call-poly <userlib>:"Valid Path__ogtk.vi"("path"=w354) -> ("valid"=w357:bool)
        n150 = Compound Arithmetic op=AND(w356, w357) -> (w355:bool)
        n151 = case shown="True" w355 {
          tunnel: w354 -> [w369 w373]
          tunnel: [w369 w372] -> w353
          tunnel: w351 -> [w368 w371]
          tunnel: [w368 w370] -> w345
          frame False {
          }
          frame True {
            n152 = while {
              shift-right: [w380] -> w372
              shift-left: w373 -> [w379]
              shift-right: [w376] -> w370
              shift-left: w371 -> [w377]
              stop <- w375 stop-if-true
              n153 = call-poly <userlib>:"File Exists__ogtk.vi"("file path"=w379) -> ("is directory"=w375:bool)  [unwired: 6 in, 1 out]
              n154 = Strip Path(path=w379) -> (stripped path=w378:path, name=w374:string)
              n155 = Select(t=w377, s=w375, f=w374) -> (s? t:f=w376:string)
              n156 = Select(t=w379, s=w375, f=w378) -> (s? t:f=w380:path)
            }
          }
        }
        n157 = case shown="\"\"" w345 {
          selector: w345 -> [w381 _]
          tunnel: [w381 w382] -> w346
          frame Default {
          }
          frame "" {
            n158 = Get Date/Time In Seconds() -> (seconds since 1Jan1904=w384:timestamp)
            n159 = Format Into String(format string="%<%Y%m%d_%H%M%S>T", w384) -> (resulting string=w382:string)  [unwired: 2 in, 1 out]
          }
        }
        n160 = call-poly <userlib>:"Strip Path Extension__ogtk.vi"("path"=w345) -> ("root"=w347:string, "extension"=w350:string)
        n161 = case shown="\"xml\"" w350 {
          tunnel: w349 -> [_ _ w367]
          tunnel: [enum16{"Plain text", "XML"}."XML" ("report format") enum16{"Plain text", "XML"}."Plain text" ("report format") w367] -> w348
          tunnel: w347 -> [w362 w364 _]
          tunnel: w346 -> [_ _ w366]
          tunnel: [w362 w364 w366] -> w344
          frame "xml" {
          }
          frame "txt" {
          }
          frame Default {
          }
        }
        n162 = Bundle By Name(cluster=w358, "Output Folder"=w353, "Report name"=w344, "report format"=w348) -> (w352:T4)
        n163 = call <vilib>:"Add State(s) to Queue__jki_lib_state_machine.vi"("State(s) in (\"\")"=w361) -> ("States Out"=w360:string)  [unwired: 14 in]
      }
      frame "Action: Find All Defined Tests" {
        n164 = Unbundle By Name(w394) -> ("Test Runner"=w390:refnum<class "Test Runner.lvclass">, "Source Folder"=w389:path)
        n165 = call-dynamic "Write Directory to search.vi"("error in (no error)"=w387, "Directory to search"=w389, "Test Runner in"=w390) -> ("error out"=w388:errorcluster, "Test Runner out"=w391:refnum<class "Test Runner.lvclass">)  [unwired: 7 in]
        n166 = call-dynamic "Discover Tests.vi"("error in (no error)"=w388, "Inspect Recursively (T)"="Inspect Recursively", "Test Runner in"=w391) -> ("error out"=w386:errorcluster, "Test Runner out"=w392:refnum<class "Test Runner.lvclass">)  [unwired: 7 in]
        n167 = Bundle By Name(cluster=w394, "Test Runner"=w392) -> (w393:T4)
        n168 = call <vilib>:"Add State(s) to Queue__jki_lib_state_machine.vi"("State(s) in (\"\")"=w396) -> ("States Out"=w395:string)  [unwired: 14 in]
      }
      frame "Action: Reset" {
        n169 = Unbundle By Name(w405) -> ("Test Runner"=w401:refnum<class "Test Runner.lvclass">, "Source Folder"=w400:path)
        n170 = call-dynamic "Write Directory to search.vi"("error in (no error)"=w398, "Directory to search"=w400, "Test Runner in"=w401) -> ("error out"=w399:errorcluster, "Test Runner out"=w402:refnum<class "Test Runner.lvclass">)  [unwired: 7 in]
        n171 = call-dynamic "Discover Tests.vi"("error in (no error)"=w399, "Test Runner in"=w402) -> ("error out"=w397:errorcluster, "Test Runner out"=w403:refnum<class "Test Runner.lvclass">)  [unwired: 8 in]
        n172 = Bundle By Name(cluster=w405, "Test Runner"=w403) -> (w404:T4)
        n173 = call <vilib>:"Add State(s) to Queue__jki_lib_state_machine.vi"("State(s) in (\"\")"=w407) -> ("States Out"=w406:string)  [unwired: 14 in]
      }
      frame "Action: Run Selected Tests" {
        n174 = Unbundle By Name(w415) -> ("Test Runner"=w417:refnum<class "Test Runner.lvclass">)
        n175 = property on="Defined Tests" class="LstBox (strict)"() -> ("Value"=w409:i32[])  [unwired: 2 in, 2 out]
        n176 = call-dynamic "Read Test VIs.vi"("Test Runner in"=w417) -> ("Test VIs"=w411:path[], "Test Runner out"=w413:refnum<class "Test Runner.lvclass">)  [unwired: 8 in, 1 out]
        n177 = Empty Array?(array=w409) -> (empty?=w408:bool)
        n178 = case shown="False" w408 {
          tunnel: w411 -> [w424 _]
          tunnel: [w423 _] -> w410
          tunnel: w409 -> [w422 _]
          frame False {
            n179 = call-poly <userlib>:"Delete Elements from Array__ogtk.vi"("indices"=w422, "array"=w424) -> ("array w/ subset deleted"=w423:path[])  [unwired: 8 in, 1 out]
          }
          frame True {
          }
        }
        n180 = call "Write Excluded Tests.vi"("Excluded Tests"=w410, "Test Runner in"=w413) -> ("Test Runner out"=w412:refnum<class "Test Runner.lvclass">)  [unwired: 8 in, 1 out]
        n181 = call-dynamic "Execute Tests.vi"("error in (no error)"=w419, "Test Runner in"=w412) -> ("error out"=w418:errorcluster, "Test Runner out"=w416:refnum<class "Test Runner.lvclass">)  [unwired: 8 in]
        n182 = Bundle By Name(cluster=w415, "Test Runner"=w416) -> (w414:T4)
        n183 = call <vilib>:"Add State(s) to Queue__jki_lib_state_machine.vi"("State(s) in (\"\")"=w421) -> ("States Out"=w420:string)  [unwired: 14 in]
      }
      frame "Action: Complete Run" {
        n184 = call <vilib>:"Add State(s) to Queue__jki_lib_state_machine.vi"("State(s) in (\"\")"=w428) -> ("States Out"=w427:string)  [unwired: 14 in]
      }
      frame "Action: Prepare Run" {
        n185 = Unbundle By Name(w435) -> ("Output Folder"=w442:path, "Report name"=w443:string, "report format"=w445:enum16{"Plain text", "XML"}, "Verbose"=w444:bool)  [unwired: 1 out]
        n186 = Unbundle By Name(w435) -> ("Interactive"=w429:bool, "Test Runner"=w436:refnum<class "Test Runner.lvclass">, "Source Folder"=w434:path)
        n187 = case shown="\"Plain text\", Default" w445 {
          tunnel: [w450 w457] -> w437
          tunnel: w444 -> [w448 w456]
          tunnel: w443 -> [w452 w463]
          tunnel: w442 -> [w453 w460]
          tunnel: [w449 w459] -> w438
          frame "Plain text", Default {
            n188 = call-poly <userlib>:"Convert File Extension__ogtk.vi"("new ending (none)"="txt", "file name"=w452) -> ("new filename"=w454:string)  [unwired: 1 out]
            n189 = Build Path(base path=w453, name or relative path=w454) -> (appended path=w451:path)
            n190 = call "Create DefaultReport.vi"("Verbose"=w448, "Report Path"=w451) -> ("error out"=w450:errorcluster, "Test Report.Default out"=w449:refnum<class "Test Report.Default.lvclass">)  [unwired: 8 in]
          }
          frame "XML" {
            n191 = call-poly <userlib>:"Convert File Extension__ogtk.vi"("new ending (none)"="xml", "file name"=w463) -> ("new filename"=w461:string)  [unwired: 1 out]
            n192 = Build Path(base path=w460, name or relative path=w461) -> (appended path=w458:path)
            n193 = call "Create JUnit Report.vi"("Verbose"=w456, "Report Path"=w458) -> ("error out"=w457:errorcluster, "Test Report.JUnit out"=w459:refnum<class "Test Report.JUnit.lvclass">)  [unwired: 8 in]
          }
        }
        n194 = call "Setup Test Runner.vi"("error in (no error)"=w437, "Test Report"=w438, "Directory to search"=w434, "Test Runner in"=w436) -> ("error out"=w431:errorcluster, "Test Runner out"=w433:refnum<class "Test Runner.lvclass">)  [unwired: 6 in]
        n195 = call "Write Interactive.vi"("error in (no error)"=w431, "Interactive"=w429, "Test Runner in"=w433) -> ("error out"=w430:errorcluster, "Test Runner out"=w432:refnum<class "Test Runner.lvclass">)  [unwired: 7 in]
        n196 = Bundle By Name(cluster=w435, "Test Runner"=w432) -> (w441:T4)
        n197 = Merge Errors(w440, w430) -> (w439:errorcluster)
        n198 = call <vilib>:"Add State(s) to Queue__jki_lib_state_machine.vi"("State(s) in (\"\")"=w447) -> ("States Out"=w446:string)  [unwired: 14 in]
      }
      frame "---------- Template ----------" {
        n199 = call <vilib>:"Add State(s) to Queue__jki_lib_state_machine.vi"("State(s) in (\"\")"=w467) -> ("States Out"=w466:string)  [unwired: 14 in]
      }
    }
  }
